vi "AI N Samples FPGA.vi"() -> ()   [LabVIEW 2019]
uses:
  <vilib>/LabVIEW Targets/FPGA/RIO/BlueMoonOnboardIO/nicrio_cRIO-BlueMoonOnboardAi_VoltageRange.ctl
  <vilib>/LabVIEW Targets/FPGA/RIO/BlueMoonOnboardIO/nicrio_cRIO-BlueMoonOnboardAi_TerminalMod.ctl
  <vilib>/Platform/TimedLoop/XDataNode/timing_clust.ctl
  <vilib>/Platform/TimedLoop/XDataNode/nitl_modes.ctl
  <vilib>/Platform/TimedLoop/XDataNode/wakeup.ctl
  <vilib>/rvi/Emulation/niFpgaGetClockAttributes.vi
  <vilib>/rvi/Emulation/niFpgaSctlEmulationGetInTimedLoop.vi
  <vilib>/rvi/Emulation/niFpgaEmulationReportErrorSimple.vi
  <vilib>/rvi/Emulation/niFpgaCriticalErrorInLSC.vi
  <vilib>/rvi/eio/common/nirviEmuTemplateMethod_errors.vi
  <vilib>/rvi/interface/RandomDataEmulation/niFpgaRandomDataHandleErrors.vi
  <vilib>/rvi/Emulation/niFpgaProcessEmulError.vi
  <vilib>/Platform/TimedLoop/XDataNode/XDataNode.xnode
  <vilib>/eio/EIOMethodNode/EIOMethodNode.xnode
  <vilib>/rvi/DataTransferAndStorage/Container/XNode/niFpgaContainer.xnode
  <vilib>/rvi/interface/RandomDataEmulation/nirviRandomDataFpgaReadWriteTemplate.vi
  <vilib>/Platform/TimedLoop/XDataNode/XDNodeRunTimeDep.lvlib
panel:
  in  "A?B":bool
  in  "Sample Number":u32 format="%.0p"
  in  "Channel Number [i + 1]":u8
  in  "Terminal Mode [i + 1]":T1=1 items=["DIFF", "RSE"]
  in  "Voltage Range [i + 1]":T2 items=["+/- 10V", "+/- 5V", "+/- 2V", "+/- 1V"]
  in  "Sample time":u32 format="%.0p"
  in  "Start":bool
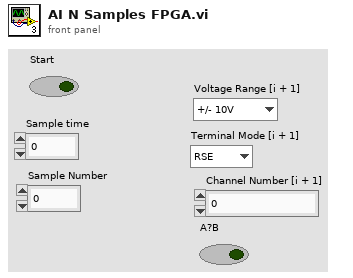
[diagram p1: front panel]
types:
  T1 = typedef "nicrio_cRIO-BlueMoonOnboardAi_TerminalMod.ctl" = u8
  T2 = typedef "nicrio_cRIO-BlueMoonOnboardAi_VoltageRange.ctl" = u8
  T3 = typedef "XDNodeRunTimeDep.lvlib/timing_clust.ctl" = cluster{"Expected End [f-1]":u64, "Actual End [f-1]":u64, "Finished Late? [f-1]":bool, "Expected End [i-1]":u64, "Actual End [i-1]":u64, "Finished Late? [i-1]":bool, "Expected Start [i]":u64, "Actual Start [i]":u64, "Expected Start [f]":u64, "Actual Start [f]":u64, "Source Name":string, "Structure Name":string, "Period":i64, "Deadline":i64, "Offset":i64, "Start":i64, "Priority":i32, "Timeout":i32, "Mode":T4, "Wakeup Reason":T5, "Error":errorcluster, "Source Type":string, "Secondary Source Type":string, "Global End Time":u64, "Global Start Time":u64, "Frame Duration":u64, "Iteration Duration":u64, "Assigned CPU":i32, "I/O Scan Engine Mode":u32}
  T4 = typedef "XDNodeRunTimeDep.lvlib/nitl_modes.ctl" = enum32{"No Change", "Process missed periods, maintain original phase", "Discard missed periods, maintain original phase", "Process missed periods, ignore original phase", "Discard missed periods, ignore original phase"}
  T5 = typedef "XDNodeRunTimeDep.lvlib/wakeup.ctl" = enum32{"Normal", "Aborted", "Asynchronous wakeup", "Timing source error", "Timed loop error", "Timeout"}
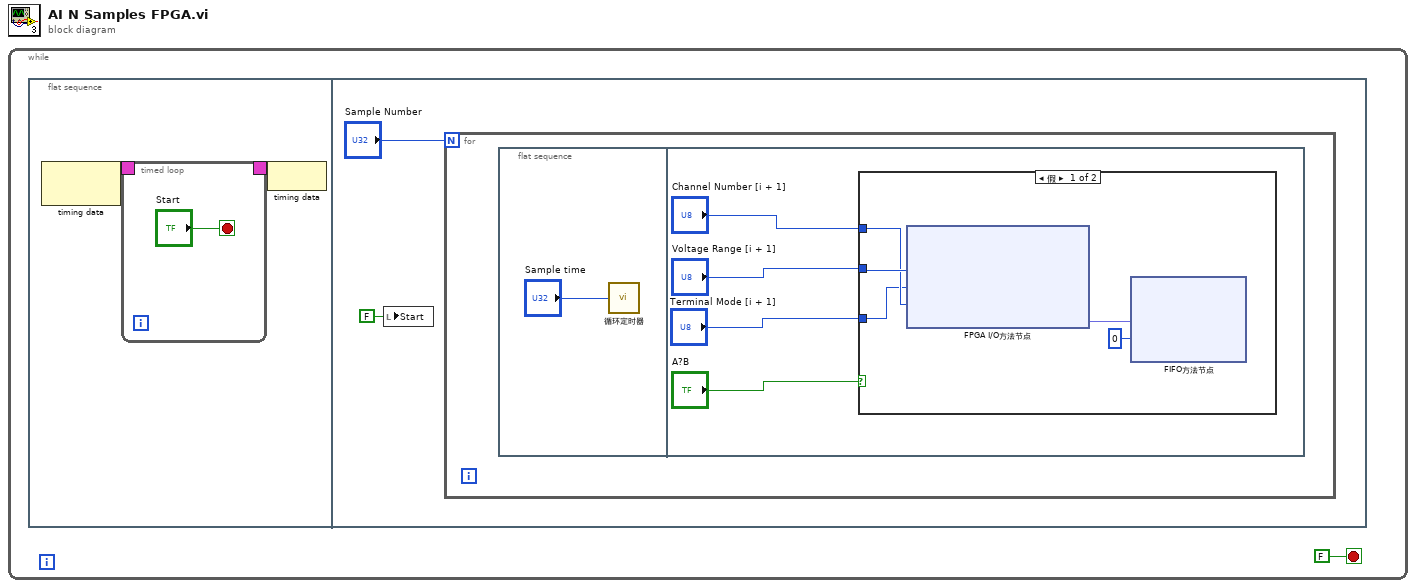
[diagram p0: block diagram]
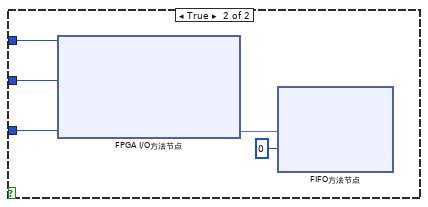
[diagram p2: hidden frame]
diagram:
  n1 = while {
    stop <- FALSE stop-if-true
    n2 = flat-sequence {
      frame #0 {
        n3 = node-c288() -> (w3:T3)  [unwired: 1 in]
        n4 = timed-loop {
          timing: w3 -> [_]
          timing-out: [_] -> w2
          stop <- "Start" stop-if-true
        }
        n5 = node-c288(w2) -> ()
      }
      frame #1 {
        n6 = local write "Start"(FALSE ("Start")) -> ()
        n7 = for {
          N: "Sample Number" -> [_]
          n8 = flat-sequence {
            frame #0 {
              n9 = call "循环定时器"("Count(uSec)"="Sample time") -> ()  [unwired: 1 out]
            }
            frame #1 {
              n10 = case shown="假" "A?B" {
                tunnel: "Voltage Range [i + 1]" -> [w20 w25]
                tunnel: "Terminal Mode [i + 1]" -> [w18 w24]
                tunnel: "Channel Number [i + 1]" -> [w19 w23]
                frame False {
                  n11 = xnode "FPGA I/O方法节点"("Voltage Range [i + 1]"=w20, "Terminal Mode [i + 1]"=w18, "Channel Number [i + 1]"=w19) -> ("Data [i]"=w17:fxp<+/-,24,5>)  [unwired: 1 in, 1 out]
                  n12 = xnode ("FIFO方法节点")("元素"=w17, "超时"=0) -> ()  [unwired: 1 in, 2 out]
                }
                frame True {
                  n13 = xnode "FPGA I/O方法节点"("Voltage Range [i + 1]"=w25, "Terminal Mode [i + 1]"=w24, "Channel Number [i + 1]"=w23) -> ("Data [i]"=w22:fxp<+/-,24,5>)  [unwired: 1 in, 1 out]
                  n14 = xnode ("FIFO方法节点")("元素"=w22, "超时"=0) -> ()  [unwired: 1 in, 2 out]
                }
              }
            }
          }
        }
      }
    }
  }
